vi "PanelClose.vi"(8 "error in (no error)":errorcluster, 11 "Module in":refnum<class "Module.lvclass">) -> (0 "error out":errorcluster, 3 "Module out":refnum<class "Module.lvclass">)   [LabVIEW 2025, in "Module.lvlib" / "Module.lvclass"]
uses:
  Module.lvclass
  Msg.ctl
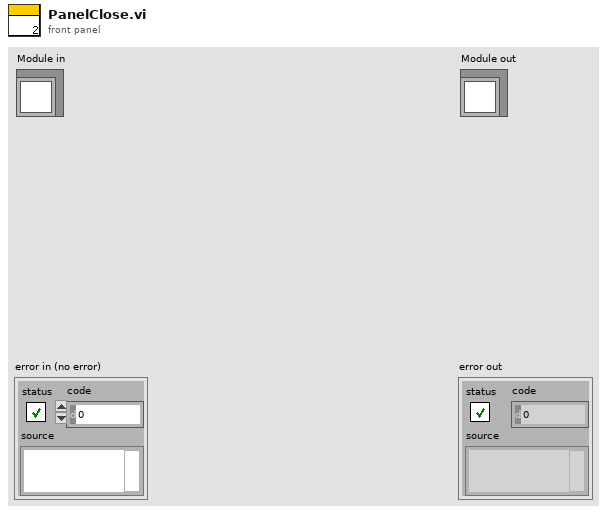
[diagram p1: front panel]
types:
  T1 = typedef "Msg.ctl" = string
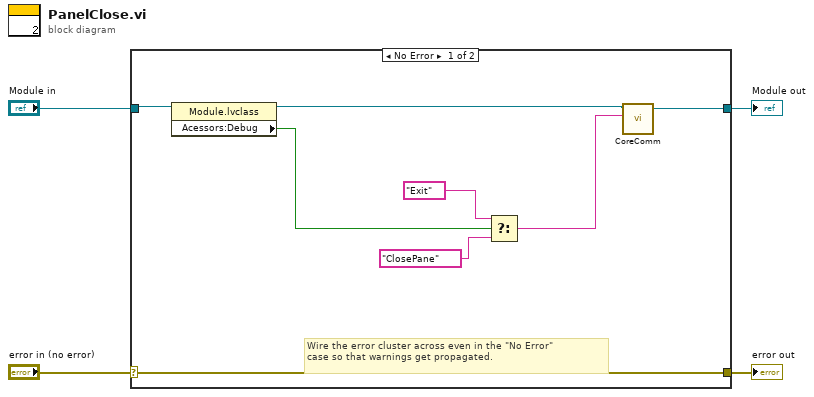
[diagram p0: block diagram]
diagram:
  n1 = case shown="No Error" "error in (no error)" {
    selector: "error in (no error)" -> [w12 w14]
    tunnel: [w12 w14] -> w3
    tunnel: [w6 w13] -> w1
    tunnel: "Module in" -> [w8 w13]
    frame No Error {
      # "Wire the error cluster across even in the \"No Error\"\ncase so that warnings get propagated."
      n2 = property class="Module.lvclass"(reference=w8) -> (reference out=w7:refnum<class "Module.lvclass">, "Acessors:Debug"=w9:bool)  [unwired: 1 in, 1 out]
      n3 = Select(t=T1 "Exit" ("Msg"), s=w9, f=T1 "ClosePane" ("Msg")) -> (s? t:f=w5:T1)
      n4 = call-dynamic "CoreComm.vi"("Msg"=w5, "Module in"=w7) -> ("Module out"=w6:refnum<class "Module.lvclass">)  [unwired: 8 in, 1 out]
    }
    frame Error {
    }
  }
  "error out" <- w3
  "Module out" <- w1
